vi "VCS Activate Position Marker.vi"(8 "error in (no error)":errorcluster, 9 "polarity":i32, 10 "digitalInputNumber":u16, 11 "axis in":cluster{"keyHandle":u32, "nodeId":u16}={"keyHandle"=0, "nodeId"=1}) -> (0 "error out":errorcluster, 3 "axis out":cluster{"keyHandle":u32, "nodeId":u16}={"keyHandle"=0, "nodeId"=1})   [LabVIEW 2010]
doc: "<B>VCS_ActivatePositionMarker</B> enables the digital input to position marker method."
uses:
  Resources/EposCmd.dll
  Resources/EposCmd64.dll
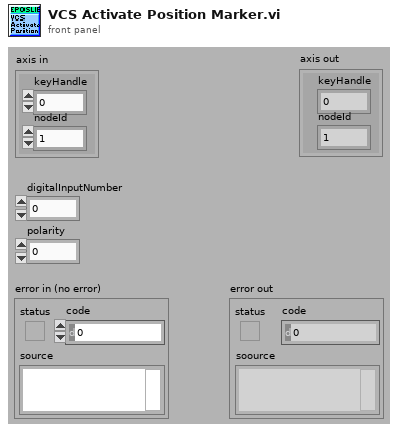
[diagram p1: front panel]
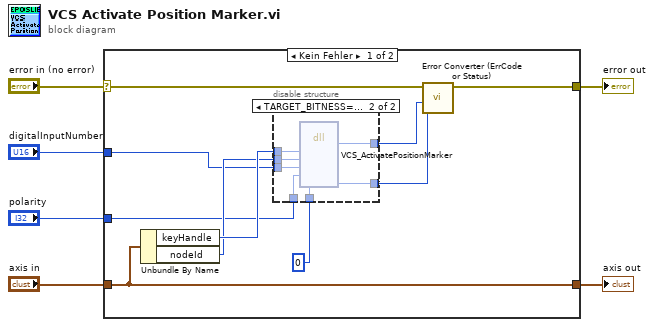
[diagram p0: block diagram]
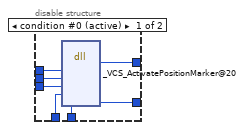
[diagram p2: hidden frame]
diagram:
  n1 = case shown="Kein Fehler" "error in (no error)" {
    selector: "error in (no error)" -> [w14 w31]
    tunnel: "axis in" -> [w16 w32]
    tunnel: [w16 w32] -> w5
    tunnel: [w15 w31] -> w4
    tunnel: "digitalInputNumber" -> [w11 _]
    tunnel: "polarity" -> [w10 _]
    frame No Error {
      n2 = Unbundle By Name(w16) -> ("keyHandle"=w13:u32, "nodeId"=w12:u16)
      n3 = disable-structure shown="TARGET_BITNESS==64" {
        disable-tunnel: w13 -> [w23 w30]
        disable-tunnel: w12 -> [w22 w29]
        disable-tunnel: w11 -> [w21 w28]
        disable-tunnel: w10 -> [w20 w27]
        disable-tunnel: u32 0 ("pErrorCode") -> [w19 w26]
        disable-tunnel: [w18 w25] -> w8
        disable-tunnel: [w17 w24] -> w7
        frame condition #0 (active) {
          n4 = dll-call lib="C:/Sources/LabView/maxon EPOS/Resources/EposCmd.*" fn="_VCS_ActivatePositionMarker@20"("KeyHandle"=w23, "NodeId"=w22, "DigitalInputNumber"=w21, "Polarity"=w20, "pErrorCode"=w19) -> (w17:i32, "pErrorCode"=w18:u32)  [unwired: 7 in, 2 out]
        }
        frame condition #1 {
          n5 = dll-call lib="C:/setup/Resources/EposCmd64.*" fn="VCS_ActivatePositionMarker" ("EposCmd.dll:_VCS_ActivatePositionMarker@20")("KeyHandle"=w30, "NodeId"=w29, "DigitalInputNumber"=w28, "Polarity"=w27, "pErrorCode"=w26) -> ("Rückgabetyp"=w24:i32, "pErrorCode"=w25:u32)  [unwired: 7 in, 2 out]
        }
      }
      n6 = call "Error Converter (ErrCode or Status).vi"("error code"=w8, "return type"=w7, "error in (no error)"=w14) -> ("error out"=w15:errorcluster)  [unwired: 7 in]
    }
    frame Error {
    }
  }
  "error out" <- w4
  "axis out" <- w5
